vi "readFromXML.vi"(8 "error in (no error)":errorcluster, 10 "XML in":string, 11 "OffsetDef in":refnum<class "OffsetDef.lvclass">) -> (0 "error out":errorcluster, 3 "OffsetDef out":refnum<class "OffsetDef.lvclass">)   [LabVIEW 2014, in "TCSDataDefinitions.lvlib" / "TCSCommand.lvlib" / "OffsetCommands.lvlib" / "OffsetDef.lvclass"]
uses:
  OffsetDef.lvclass
  Enumerations/Num1Types.ctl
  Enumerations/OffsetType.ctl
  <userlib>/Common/UnitsAndXML/FlattenItemWithUnitToXML/FlattenTimeToXML/TimeUnit.ctl
  <userlib>/Common/UnitsAndXML/FlattenItemWithUnitToXML/FlattenPlaneAngleToXML/PlaneAngleUnit.ctl
  OffsetDef.lvclass/OffsetDef.ctl
  <userlib>/Common/UnitsAndXML/UnitsAndXML.lvlib
  <userlib>/Common/XML/XMLParser/XMLParser.lvclass
  OffsetCommands.lvlib
panel:
  out "offsetType":T1
  out "num1":T2
  out "off2":dbl[unit]
  out "off1":dbl[unit]
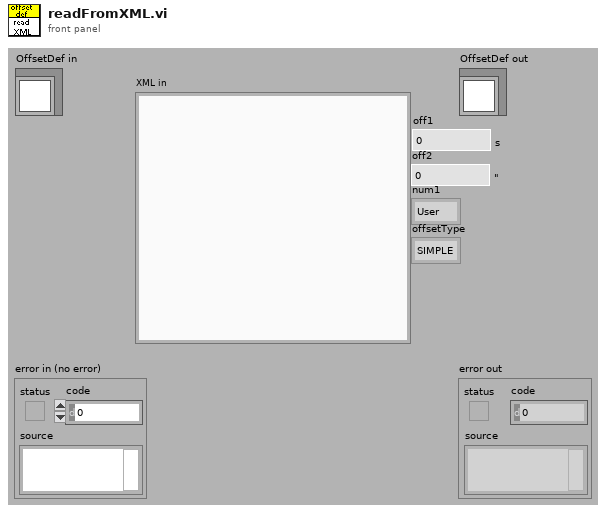
[diagram p1: front panel]
types:
  T1 = typedef "TCSDataDefinitions.lvlib/TCSCommand.lvlib/OffsetCommands.lvlib/OffsetType.ctl" = enum16{"SIMPLE", "TPLANE", "PA"}
  T2 = typedef "TCSDataDefinitions.lvlib/TCSCommand.lvlib/OffsetCommands.lvlib/Num1Types.ctl" = enum16{"User", "Handset"}
  T3 = typedef "UnitsAndXML.lvlib/PlaneAngleUnit.ctl" = enum16{"rad", "deg", "'", "\""}
  T4 = typedef "UnitsAndXML.lvlib/TimeUnit.ctl" = enum16{"s", "d", "h", "min", "a"}
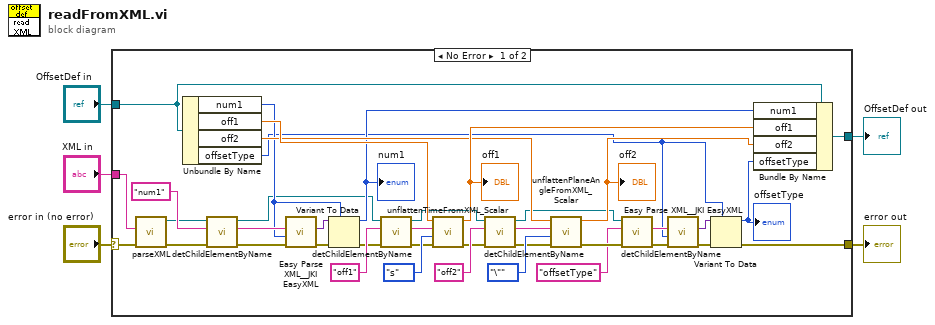
[diagram p0: block diagram]
diagram:
  n1 = case shown="No Error" "error in (no error)" {
    selector: "error in (no error)" -> [w40 w46]
    tunnel: [w27 w45] -> w3
    tunnel: "OffsetDef in" -> [w28 w45]
    tunnel: "XML in" -> [w44 _]
    tunnel: [w11 w46] -> w1
    frame No Error {
      n2 = call <userlib>:"parseXML.vi"("error in (no error)"=w40, "XMLString in"=w44) -> ("error out"=w41:errorcluster, "Element out"=w9:refnum<class "XMLParser.lvclass">)  [unwired: 8 in]
      n3 = Unbundle By Name(w28) -> ("num1"=w18:T2, "off1"=w24:dbl[unit], "off2"=w23:dbl[unit], "offsetType"=w13:T1)
      n4 = call <userlib>:"detChildElementByName.vi"("error in (no error)"=w41, "childName"="num1" ("ChildName"), "Element in"=w9) -> ("error out"=w20:errorcluster, "childXML"=w29:string, "Element out"=w8:refnum<class "XMLParser.lvclass">)  [unwired: 5 in, 1 out]
      n5 = call <vilib>:"Easy Parse XML__JKI EasyXML.vi"("error in (no error)"=w20, "LabVIEW Data (Type)"=w18, "XML String"=w29) -> ("error out"=w31:errorcluster, "LabVIEW Data"=w30:variant)  [unwired: 7 in]
      n6 = Variant To Data(error in=w31, type=w18, Variant=w30) -> (data=w17:T2, error out=w19:errorcluster)
      "num1" <- w17
      n7 = call <userlib>:"detChildElementByName.vi"("error in (no error)"=w19, "childName"="off1" ("ChildName"), "Element in"=w8) -> ("error out"=w37:errorcluster, "childXML"=w39:string, "Element out"=w7:refnum<class "XMLParser.lvclass">)  [unwired: 5 in, 1 out]
      n8 = call <userlib>:"unflattenTimeFromXML_Scalar.vi"("error in (no error)"=w37, "timeUnitInXML"=TimeUnit."s", "xmlString"=w39, "timeForType"=w24) -> ("error out"=w36:errorcluster, "time"=w26:dbl[unit])  [unwired: 6 in]
      "off1" <- w26
      n9 = call <userlib>:"detChildElementByName.vi"("error in (no error)"=w36, "childName"="off2" ("ChildName"), "Element in"=w7) -> ("error out"=w33:errorcluster, "childXML"=w35:string, "Element out"=w6:refnum<class "XMLParser.lvclass">)  [unwired: 5 in, 1 out]
      n10 = call <userlib>:"unflattenPlaneAngleFromXML_Scalar.vi"("error in (no error)"=w33, "planeAngleUnitInXML"=PlaneAngleUnit."\"", "xmlString"=w35, "planeAngleForType"=w23) -> ("error out"=w32:errorcluster, "planeAngle"=w25:dbl[unit])  [unwired: 6 in]
      "off2" <- w25
      n11 = call <userlib>:"detChildElementByName.vi"("error in (no error)"=w32, "childName"="offsetType" ("ChildName"), "Element in"=w6) -> ("error out"=w10:errorcluster, "childXML"=w14:string)  [unwired: 5 in, 2 out]
      n12 = call <vilib>:"Easy Parse XML__JKI EasyXML.vi"("error in (no error)"=w10, "LabVIEW Data (Type)"=w13, "XML String"=w14) -> ("error out"=w16:errorcluster, "LabVIEW Data"=w15:variant)  [unwired: 7 in]
      n13 = Variant To Data(error in=w16, type=w13, Variant=w15) -> (data=w12:T1, error out=w11:errorcluster)
      "offsetType" <- w12
      n14 = Bundle By Name(cluster=w28, "num1"=w17, "off1"=w26, "off2"=w25, "offsetType"=w12) -> (w27:refnum<class "OffsetDef.lvclass">)
    }
    frame Error {
    }
  }
  "error out" <- w1
  "OffsetDef out" <- w3
